vi "generateVinVout.vi"(10 "interleaved array":dbl[](array[numeric])) -> (1 "CHB":string, 2 "CHA":string)   [LabVIEW 2010]
panel:
  out "decimated array 2":dbl[](array[numeric])
  out "decimated array":dbl[](array[numeric])
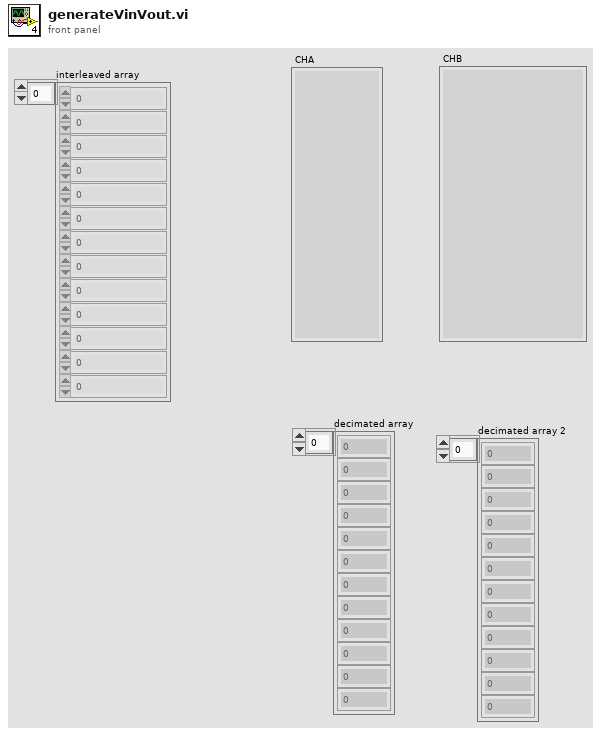
[diagram p1: front panel]
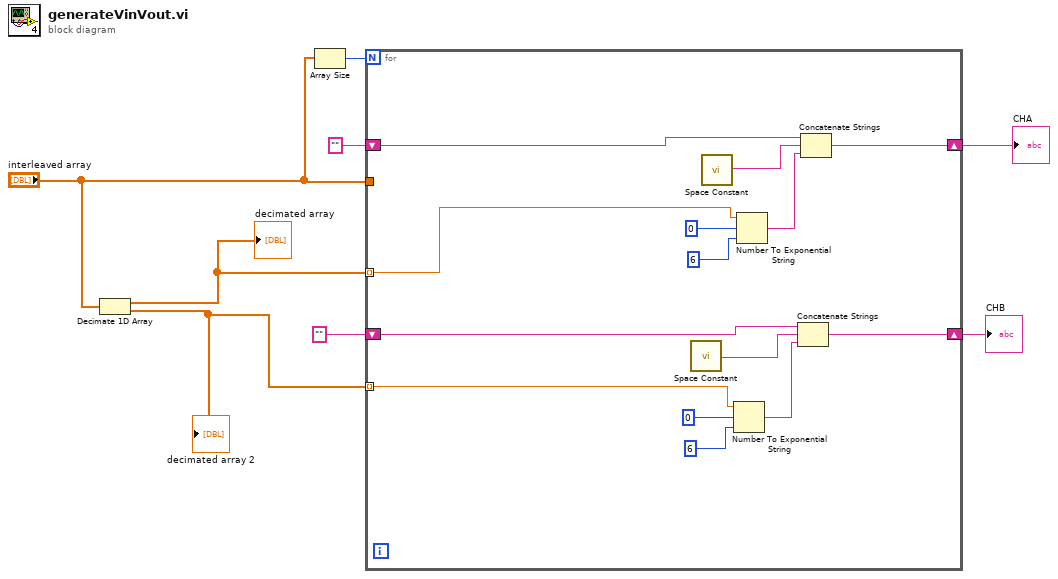
[diagram p0: block diagram]
diagram:
  n1 = Decimate 1D Array("interleaved array") -> (w2:dbl[], w1:dbl[])
  "decimated array" <- w2
  "decimated array 2" <- w1
  n2 = Array Size(array="interleaved array") -> (size(s)=w8:i32)
  n3 = for {
    N: w8 -> [_]
    shift-right: [w22] -> w6
    shift-left: "" -> [w20]
    tunnel: "interleaved array" -> [_]
    shift-right: [w14] -> w5
    shift-left: "" -> [w13]
    tunnel: w2 -> [w12] mode=indexing
    tunnel: w1 -> [w11] mode=indexing
    n4 = call <vilib>:"Space Constant.vi"() -> ("String"=w9:string)
    n5 = call <vilib>:"Space Constant.vi"() -> ("String"=w10:string)
    n6 = Number To Exponential String(number=w11, precision (6)=i16 6, 3:i16 0 ("width (-)")) -> (E-format string=w17:string)  [unwired: 1 in]
    n7 = Number To Exponential String(number=w12, precision (6)=i16 6, 3:i16 0 ("width (-)")) -> (E-format string=w21:string)  [unwired: 1 in]
    n8 = Concatenate Strings(w13, w9, w17) -> (w14:string)
    n9 = Concatenate Strings(w20, w10, w21) -> (w22:string)
  }
  "CHA" <- w6
  "CHB" <- w5
